vi "main.vi"() -> ()   [LabVIEW 2018]
uses:
  <vilib>/addons/database/Connection.llb/DB Tools Open Connec (Path).vi
  <vilib>/addons/database/NI_Database_API.lvlib
panel:
  out "温度":dbl
  out "负责人信息":T1
  out "疫苗信息":T2 {"生产日期" format="%<%Y/%m/%d>T"}
  in  "CYJ":bool
  in  "比例尺":i16(slide) scale=10.0..18.0
  in  "地图":refnum<k7>(container) caption="网页浏览器"
  out "经度":string
  out "纬度":string
  in  "stop":bool caption="停止"
  out "时间":timestamp format="%<%x %H:%M:%S>T"
  out "掉线":bool
  # "疫苗冷链储运监控系统\n             VACCINE  COLD-CHAIN TRANSPORTATION MONITORING SYSTEM"
  # "智能装备学院\n南工自动152"
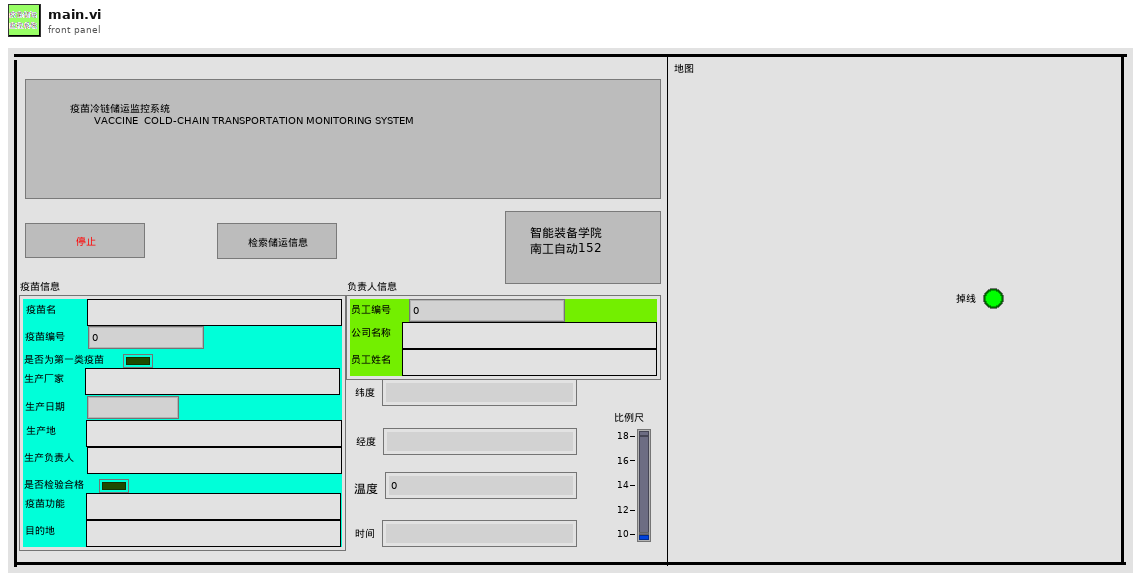
[diagram p1: front panel]
types:
  T1 = typedef "人员信息.ctl" = cluster{"员工编号":i32, "公司名称":string, "员工姓名":string}
  T2 = typedef "疫苗信息.ctl" = cluster{"疫苗名":string, "疫苗编号":i32, "是否为第一类疫苗":bool, "生产厂家":string, "生产日期":timestamp, "生产地":string, "生产负责人":string, "是否检验合格":bool, "疫苗功能":string, "目的地":string}
  T3 = typedef "NI_Database_API.lvlib/Conn ObjectReference.ctl" = refnum<k1>
  T4 = typedef "储运信息.ctl" = cluster{"纬度":sgl, "经度":sgl, "温度":sgl, "负责人":i32, "区域":string, "记录时间":timestamp}
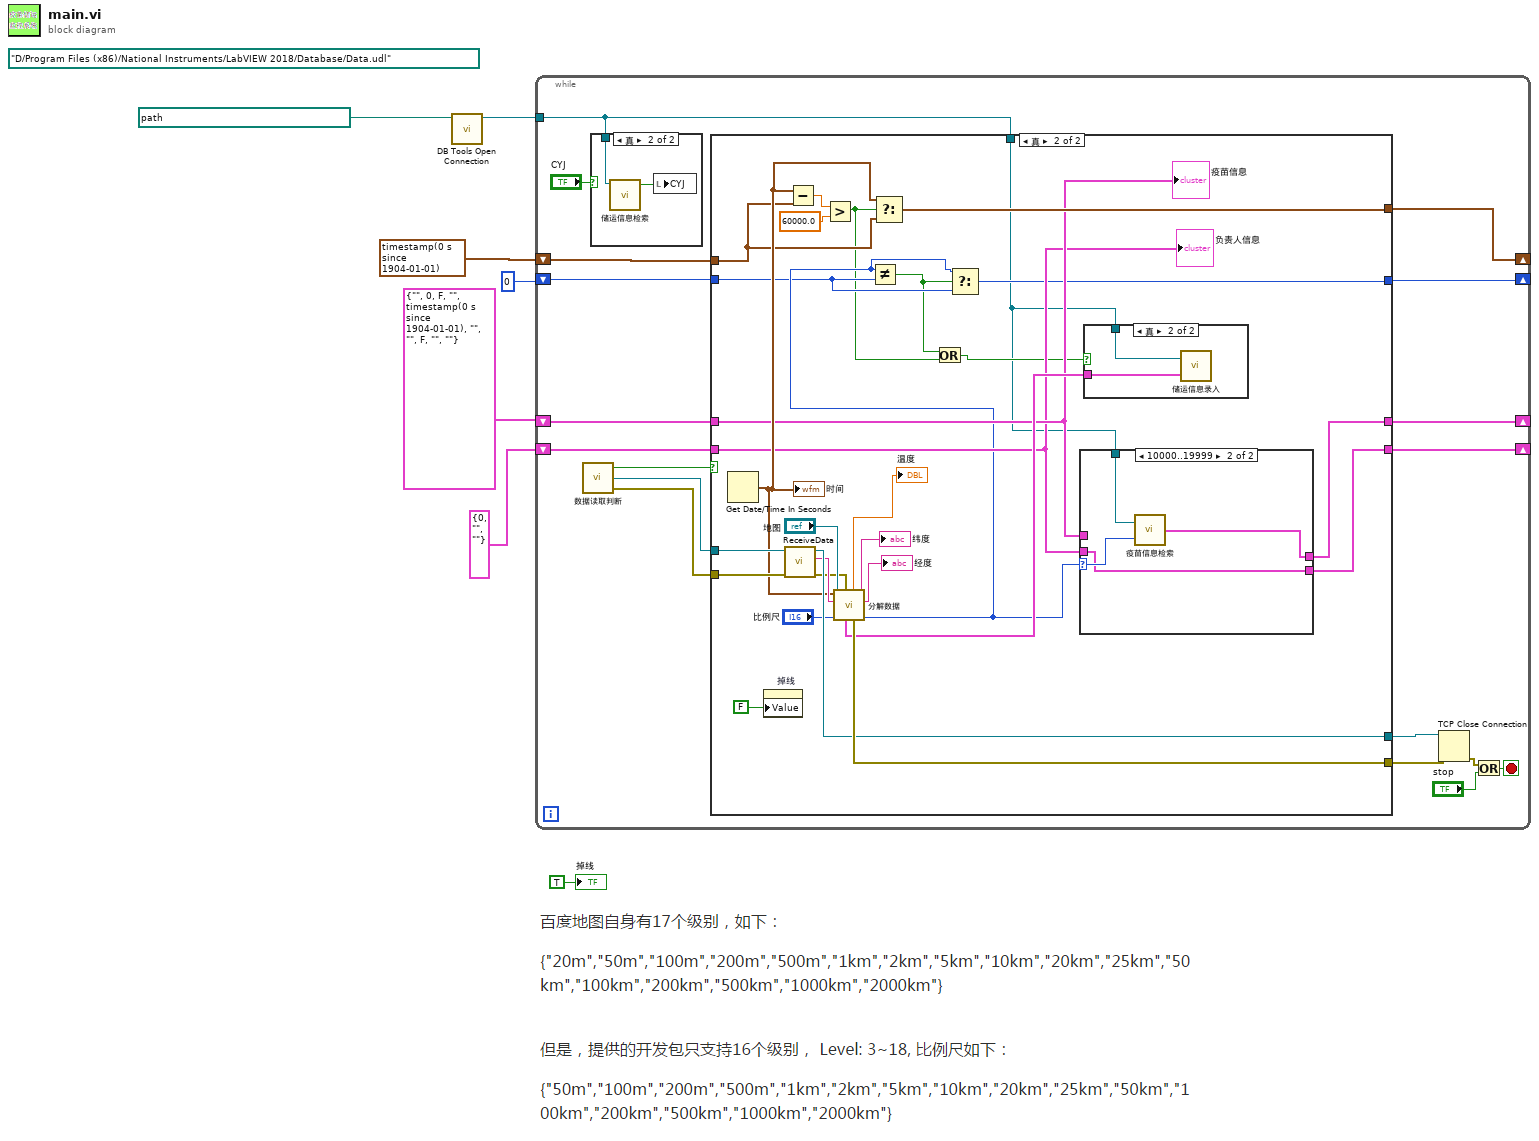
[diagram p0: block diagram]
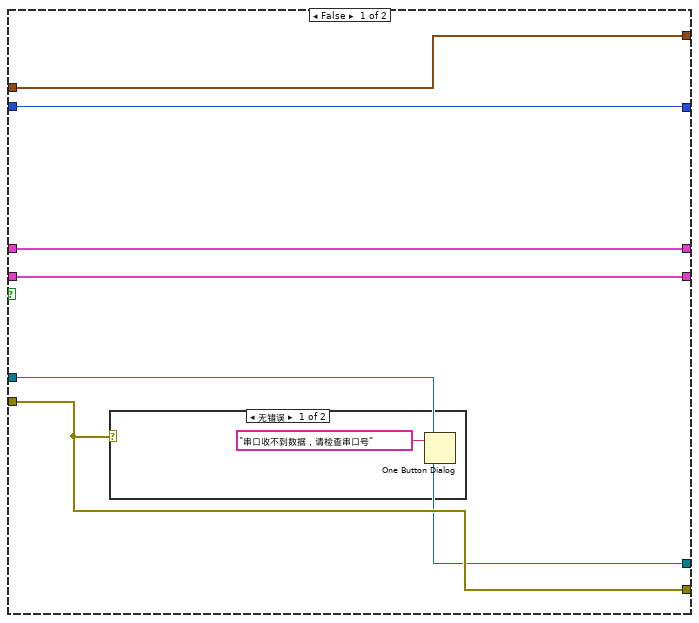
[diagram p3: hidden frame]
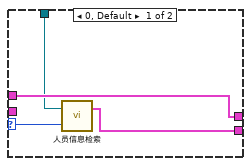
[diagram p6: hidden frame]
diagram:
  (unwired) path "D:/Program Files (x86)/National Instruments/LabVIEW 2018/Database/Data.udl" ("路径")
  n1 = call-poly <vilib>:"DB Tools Open Connection.vi"("connection information"=path "D:/2019毕业设计/Code/GPData.udl" ("路径")) -> ("connection reference"=w6:T3)  [unwired: 7 in, 1 out]
  n2 = while {
    tunnel: w6 -> [w11]
    shift-right: [w10] -> _
    shift-left: T2 {"疫苗名"="", "疫苗编号"=0, "是否为第一类疫苗"=FALSE, "生产厂家"="", "生产日期"=timestamp(0 s since 1904-01-01), "生产地"="", "生产负责人"="", "是否检验合格"=FALSE, "疫苗功能"="", "目的地"=""} ("簇") -> [w16]
    shift-right: [w14] -> _
    shift-left: T1 {"员工编号"=0, "公司名称"="", "员工姓名"=""} ("负责人数据") -> [w15]
    shift-right: [w12] -> _
    shift-left: timestamp(0 s since 1904-01-01) ("时间标识") -> [w13]
    shift-right: [w8] -> _
    shift-left: 0 -> [w9]
    stop <- w25 stop-if-true
    n3 = call "数据读取判断.vi"() -> ("error out"=w21:errorcluster, "connection ID"=w22:refnum<k5>, "判断错误"=w23:bool)
    n4 = case shown="真" "CYJ" {
      tunnel: w11 -> [_ w27]
      frame False {
      }
      frame True {
        n5 = call "储运信息检索.vi"("connection reference"=w27) -> ("布尔"=w26:bool)  [unwired: 3 in, 2 out]
        n6 = local write "CYJ"(w26) -> ()
      }
    }
    n7 = case shown="真" w23 {
      tunnel: w21 -> [w33 w63]
      tunnel: [w32 w61] -> w18
      tunnel: [w33 w62] -> w20
      tunnel: w22 -> [w32 w60]
      tunnel: w11 -> [_ w35]
      tunnel: [w31 w52] -> w10
      tunnel: w16 -> [w31 w44]
      tunnel: w15 -> [w30 w43]
      tunnel: [w30 w51] -> w14
      tunnel: w13 -> [w29 w47]
      tunnel: [w29 w46] -> w12
      tunnel: w9 -> [w28 w39]
      tunnel: [w28 w41] -> w8
      frame False {
        n8 = case shown="无错误" w33 {
          frame No Error {
            n9 = One Button Dialog(message="串口收不到数据，请检查串口号" ("消息")) -> ()  [unwired: 1 in, 1 out]
          }
          frame Error {
          }
        }
      }
      frame True {
        n10 = Get Date/Time In Seconds() -> (seconds since 1Jan1904=w48:timestamp)
        "时间" <- w48
        n11 = property on="掉线" class="Bool (严格)"("Value"=FALSE ("掉线")) -> ()  [unwired: 2 in, 2 out]
        n12 = call "ReceiveData.vi"("错误输入（无错误）"=w63, "连接ID"=w60) -> ("错误输出"=w55:errorcluster, "dataOut"=w58:string, "连接ID输出"=w61:refnum<k5>)  [unwired: 5 in, 2 out]
        n13 = Subtract(x=w48, y=w47) -> (x-y=w50:dbl)
        n14 = Greater?(x=w50, y=60000.0) -> (0:w37:bool)
        n15 = call "分解数据.vi"("error IO"=w55, "滑动杆"="比例尺", "地图"="地图", "data"=w58, "时间"=w48) -> ("uid"=w40:i16, "纬度显示"=→"经度":string, "经度显示"=→"纬度":string, "错误输出"=w62:errorcluster, "温度"=→"温度":sgl, "待写入的簇"=w45:T4)  [unwired: 1 out]
        n16 = Not Equal?(x=w40, y=w39) -> (x != y?=w38:bool)
        n17 = Select(t=w48, s=w37, f=w47) -> (s? t:f=w46:timestamp)
        n18 = Or(x=w38, y=w37) -> (x .or. y?=w36:bool)
        n19 = Select(t=w40, s=w38, f=w39) -> (s? t:f=w41:i32)
        n20 = case shown="10000..19999" w40 {
          selector: w40 -> [w69 w73]
          tunnel: [w68 w72] -> w52
          tunnel: w44 -> [w68 _]
          tunnel: w43 -> [_ w71]
          tunnel: [w67 w71] -> w51
          tunnel: w35 -> [w66 w70]
          frame 0, Default {
            n21 = call "人员信息检索.vi"("工作人员编号"=w69, "connection reference"=w66) -> ("负责人数据"=w67:T1)  [unwired: 1 out]
          }
          frame 10000..19999 {
            n22 = call "疫苗信息检索.vi"("疫苗编号"=w73, "connection reference"=w70) -> ("疫苗数据"=w72:T2)
          }
        }
        n23 = case shown="真" w36 {
          tunnel: w35 -> [_ w64]
          tunnel: w45 -> [_ w65]
          frame False {
          }
          frame True {
            n24 = call "储运信息录入.vi"("储运信息"=w65, "connection reference"=w64) -> ()  [unwired: 1 out]
          }
        }
        "疫苗信息" <- w44
        "负责人信息" <- w43
      }
    }
    n25 = TCP Close Connection(connection ID=w18, error in (no error)=w20) -> (error out=w24:errorcluster)  [unwired: 1 in, 1 out]
    n26 = Or(x=w24, y="stop") -> (x .or. y?=w25:bool)
  }
  "掉线" <- TRUE ("掉线")
